vi "Load Module.vi"(8 "error in (no error)":errorcluster) -> (0 "error out":errorcluster)   [LabVIEW 2020, in "Dummy.lvlib"]
doc: "____\nHAMPEL SOFTWARE ENGINEERING v2.6.0 (2023-12-19 10:54)"
uses:
  Dummy.lvlib
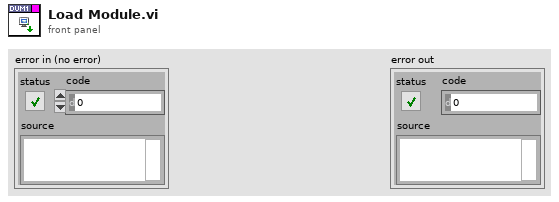
[diagram p1: front panel]
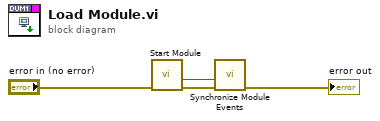
[diagram p0: block diagram]
diagram:
  n1 = call "Start Module.vi"("error in (no error)"="error in (no error)") -> ("error out"=w4:errorcluster, "Wait for Event Sync?"=w3:bool)  [unwired: 7 in, 2 out]
  n2 = call "Synchronize Module Events.vi"("error in (no error)"=w4, "Wait for Event Sync?"=w3) -> ("error out"=→"error out":errorcluster)  [unwired: 9 in]
